vi "SwissSPAD Live_Close Communication.vi"(8 "Error In":errorcluster, 11 "SwissSPAD Live Internal Variables":T1={"okCFrontPanelDevices Refnum"=refnum, "Bottom Device Refnum"=refnum, "Display Image"=refnum, "# Live Images"=0, "relative s"=0.0, "# Image Sets"=0, "Message"="", "Current Image Set"=0, "# Datasets in Series"=0, "Current Dataset"=0, "Live Mode"=FALSE, "Recording Mode"=FALSE, "Record Button"=refnum, "\nLive Button"=refnum, "SwissSPAD Live Gate Image Data Q Name"="SS2 Live Gate Data Q", "Discard First Image"=FALSE, "Image Information"={"Save ROI Only"=FALSE, "Left"=0, "Top"=0, "Right"=0, "Bottom"=0, "Use Current ROI"=FALSE}, "Image Binning Options"={"Use Image Binning"=FALSE, "X Bin"=1, "Y Bin"=1}, "Bottom FPGA Serial Number"="", "Detector PCB Version"=enum."SS2 PCB1", "# Acquisitions"=1, "10 bits"=FALSE, "Top FPGA Serial Number"="", "Top Device Refnum"=refnum, "okCFrontPanel Refnum"=refnum} {"# Acquisitions" min=1; "Image Binning Options"."Y Bin" min=1; "Image Binning Options"."X Bin" min=1}) -> (0 "Error Out":errorcluster, 3 "SwissSPAD Live Internal Variables":T1={"okCFrontPanelDevices Refnum"=refnum, "Bottom Device Refnum"=refnum, "Display Image"=refnum, "# Live Images"=0, "relative s"=0.0, "# Image Sets"=0, "Message"="", "Current Image Set"=0, "# Datasets in Series"=0, "Current Dataset"=0, "Live Mode"=FALSE, "Recording Mode"=FALSE, "Record Button"=refnum, "\nLive Button"=refnum, "SwissSPAD Live Gate Image Data Q Name"="SS2 Live Gate Data Q", "Discard First Image"=FALSE, "Image Information"={"Save ROI Only"=FALSE, "Left"=0, "Top"=0, "Right"=0, "Bottom"=0, "Use Current ROI"=FALSE}, "Image Binning Options"={"Use Image Binning"=FALSE, "X Bin"=1, "Y Bin"=1}, "Bottom FPGA Serial Number"="", "Detector PCB Version"=enum."SS2 PCB1", "# Acquisitions"=1, "10 bits"=FALSE, "Top FPGA Serial Number"="", "Top Device Refnum"=refnum, "okCFrontPanel Refnum"=refnum} {"# Acquisitions" min=1; "Image Binning Options"."Y Bin" min=1; "Image Binning Options"."X Bin" min=1})   [LabVIEW 2021]
uses:
  SwissSPAD Live_Internal Variables.ctl
  D:/UCLA Thinkpad Google Drive/LabVIEW 2021 SP1/builds/SwissSPAD Live Distribution/Opal Kelly/C# Wrapper/v5.0.2/libFrontPanel-csharp.dll
  Opal Kelly/C# Wrapper/v5.0.2/libFrontPanel-csharp.dll
  <vilib>/vision/Image Controls.llb/IMAQ Image.ctl
  SwissSPAD Live_Image ROI Information.ctl
  Phasor/Image Binning Options.ctl
  SwissSPAD Live_SSx PCB Version.ctl
  Opal Kelly/C# Wrapper/okFrontPanelC#Wrapper.lvlib
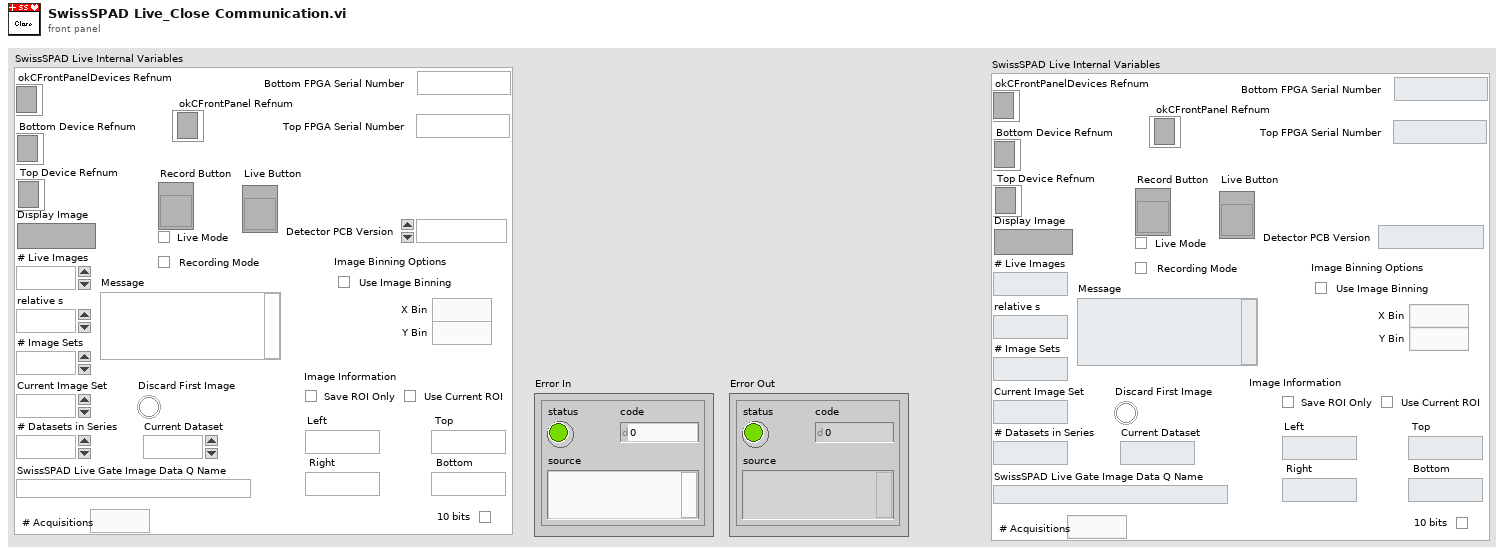
[diagram p1: front panel]
types:
  T1 = typedef "SwissSPAD Live_Internal Variables.ctl" = cluster{"okCFrontPanelDevices Refnum":refnum<k24>, "Bottom Device Refnum":refnum<k24>, "Display Image":T2, "# Live Images":i32, "relative s":dbl, "# Image Sets":i32, "Message":string, "Current Image Set":i32, "# Datasets in Series":i32, "Current Dataset":i32, "Live Mode":bool, "Recording Mode":bool, "Record Button":refnum<vi>, "\nLive Button":refnum<vi>, "SwissSPAD Live Gate Image Data Q Name":string, "Discard First Image":bool, "Image Information":T3, "Image Binning Options":T4, "Bottom FPGA Serial Number":string, "Detector PCB Version":T5, "# Acquisitions":u32, "10 bits":bool, "Top FPGA Serial Number":string, "Top Device Refnum":refnum<k24>, "okCFrontPanel Refnum":refnum<k24>}
  T2 = typedef "IMAQ Image.ctl" = refnum<image>
  T3 = typedef "SwissSPAD Live_Image ROI Information.ctl" = cluster{"Save ROI Only":bool, "Left":u16, "Top":u16, "Right":u16, "Bottom":u16, "Use Current ROI":bool}
  T4 = typedef "Image Binning Options.ctl" = cluster{"Use Image Binning":bool, "X Bin":i32, "Y Bin":i32}
  T5 = typedef "SwissSPAD Live_SSx PCB Version.ctl" = enum16{"unknown", "SS2 PCB1", "SS2 PCB2", "SS3 PCB1"}
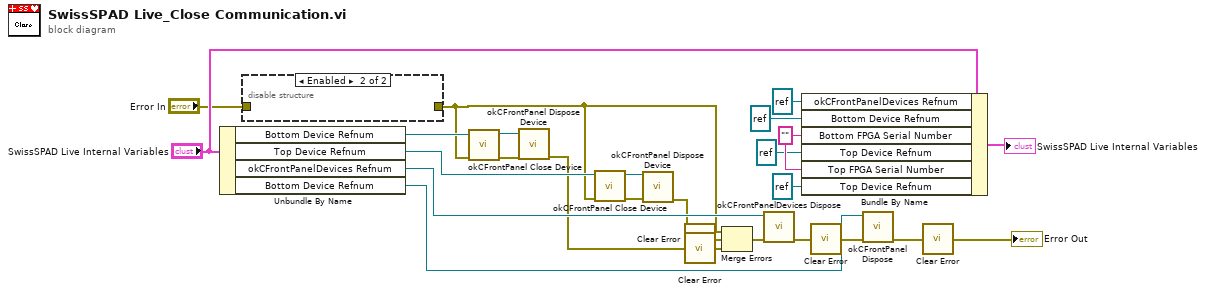
[diagram p0: block diagram]
diagram:
  w18 = "" ("Bottom FPGA Serial Number")
  n1 = Unbundle By Name("SwissSPAD Live Internal Variables") -> ("Bottom Device Refnum"=w26:refnum<k24>, "Top Device Refnum"=w25:refnum<k24>, "okCFrontPanelDevices Refnum"=w24:refnum<k24>, "Bottom Device Refnum"=w4:refnum<k24>)
  n2 = disable-structure shown="Enabled" {
    disable-tunnel: "Error In" -> [w27 _]
    disable-tunnel: [w27 _] -> w6
    frame Disabled {
    }
    frame Enabled {
    }
  }
  n3 = call "okCFrontPanel Close Device.vi"("error in (no error)"=w6, "okCFrontPanel Device Refnum"=w26) -> ("error out"=w12:errorcluster, "okCFrontPanel Refnum out"=w13:refnum<k24>)  [unwired: 8 in]
  n4 = call "okCFrontPanel Dispose Device.vi"("Error In"=w12, "okCFrontPanel Refnum"=w13) -> ("Error Out"=w11:errorcluster)  [unwired: 9 in]
  n5 = call "okCFrontPanel Close Device.vi"("error in (no error)"=w6, "okCFrontPanel Device Refnum"=w25) -> ("error out"=w10:errorcluster, "okCFrontPanel Refnum out"=w8:refnum<k24>)  [unwired: 8 in]
  n6 = call "okCFrontPanel Dispose Device.vi"("Error In"=w10, "okCFrontPanel Refnum"=w8) -> ("Error Out"=w9:errorcluster)  [unwired: 9 in]
  n7 = call "Clear Error.vi"("Error In"=w9) -> ("no Error Out"=w21:errorcluster)  [unwired: 8 in]
  n8 = call "Clear Error.vi"("Error In"=w11) -> ("no Error Out"=w14:errorcluster)  [unwired: 8 in]
  n9 = Merge Errors(w6, w21, w14) -> (w23:errorcluster)
  n10 = call "okCFrontPanelDevices Dispose.vi"("Error In"=w23, "okCFrontPanelDevices Refnum"=w24) -> ("Error Out"=w22:errorcluster)  [unwired: 9 in]
  n11 = Bundle By Name(cluster="SwissSPAD Live Internal Variables", "okCFrontPanelDevices Refnum"=refnum<k24> refnum, "Bottom Device Refnum"=refnum<k24> refnum, "Bottom FPGA Serial Number"=w18, "Top Device Refnum"=refnum<k24> refnum, "Top FPGA Serial Number"=w18, "Top Device Refnum"=refnum<k24> refnum) -> (→"SwissSPAD Live Internal Variables":T1)
  n12 = call "Clear Error.vi"("Error In"=w22) -> ("no Error Out"=w5:errorcluster)  [unwired: 8 in]
  n13 = call "okCFrontPanel Dispose.vi"("Error In"=w5, "okCFrontPanel Refnum"=w4) -> ("Error Out"=w3:errorcluster)  [unwired: 9 in]
  n14 = call "Clear Error.vi"("Error In"=w3) -> ("no Error Out"=→"Error Out":errorcluster)  [unwired: 8 in]
